vi "Drive for set feet.vi"(8 "Encoder ID":i32, 9 "Total Distance":dbl=10.0 format="%#_13g", 10 "Enum":T1(ring), 11 "Feet":dbl=10.0 format="%#_13g") -> (2 "Distance":dbl(knob) scale=0.0..10.0)   [LabVIEW 2014]
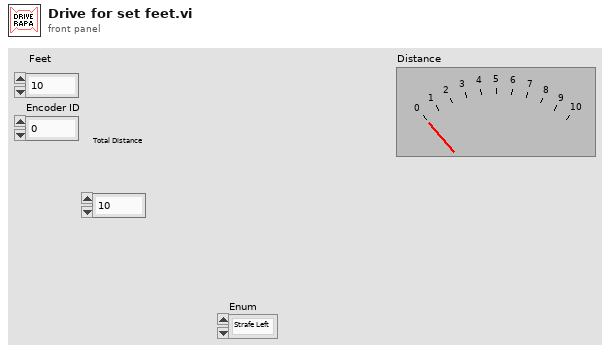
[diagram p1: front panel]
types:
  T1 = enum16{"Strafe Left", "Strafe Right", "Forwards", "Backwards"}
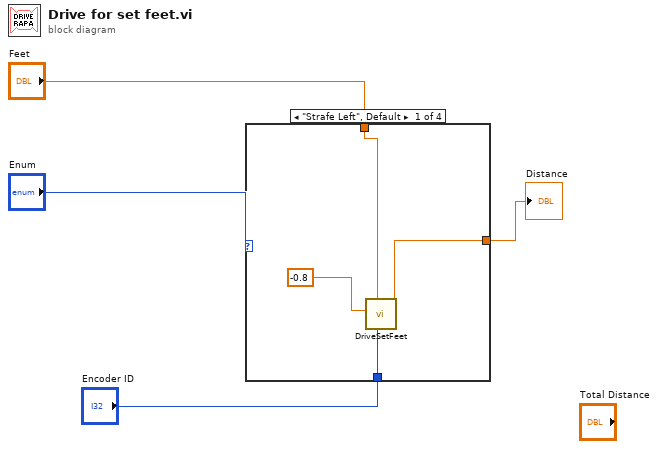
[diagram p0: block diagram]
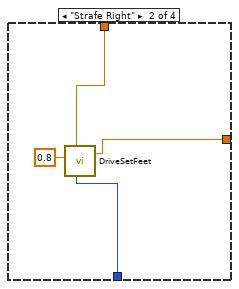
[diagram p2: hidden frame]
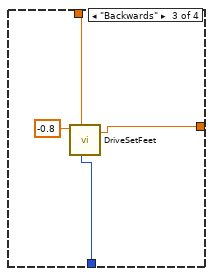
[diagram p3: hidden frame]
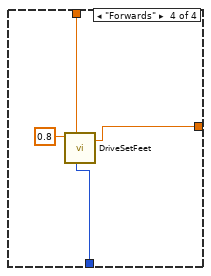
[diagram p4: hidden frame]
diagram:
  n1 = case shown="\"Strafe Left\", Default" "Enum" {
    tunnel: "Feet" -> [w7 w11 w15 w19]
    tunnel: [w6 w12 w14 w18] -> w2
    tunnel: "Encoder ID" -> [w5 w9 w13 w17]
    frame "Strafe Left", Default {
      n2 = call "DriveSetFeet.vi"("Encoder ID"=w5, "Feet"=w7, "Strafe"=-0.8) -> ("Distance"=w6:dbl)  [unwired: 3 in, 1 out]
    }
    frame "Strafe Right" {
      n3 = call "DriveSetFeet.vi"("Encoder ID"=w9, "Feet"=w11, "Strafe"=0.8) -> ("Distance"=w12:dbl)  [unwired: 3 in, 1 out]
    }
    frame "Backwards" {
      n4 = call "DriveSetFeet.vi"("Encoder ID"=w13, "Feet"=w15, "Forward/Backward"=-0.8) -> ("Distance"=w14:dbl)  [unwired: 3 in, 1 out]
    }
    frame "Forwards" {
      n5 = call "DriveSetFeet.vi"("Encoder ID"=w17, "Feet"=w19, "Forward/Backward"=0.8) -> ("Distance"=w18:dbl)  [unwired: 3 in, 1 out]
    }
  }
  "Distance" <- w2
